vi "Lab Panel V5.11.vi"() -> ()   [LabVIEW 2013] (continued)
                            n2200 = Bundle(cluster=w3959, "amps"=w3963, "volts"=w3962, "pf"=w3961) -> (w3960:cluster{"amps":dbl, "volts":dbl, "pf":dbl})
                            n2201 = local write "ON L01-2"(w3960) -> ()
                          }
                        }
                      }
                      frame #1 {
                        n2202 = Unbundle(w3968) -> ("amps"=w3967:dbl, "volts"=w3966:dbl, "pf"=w3965:dbl)
                        n2203 = case shown="True" w3969 {
                          tunnel: w3976 -> [_ w4008]
                          tunnel: w3975 -> [_ w4015]
                          tunnel: w3974 -> [_ _]
                          tunnel: w3973 -> [_ _]
                          tunnel: w3972 -> [_ w4014]
                          tunnel: w3971 -> [_ w4013]
                          tunnel: w3970 -> [_ w3978]
                          tunnel: w3967 -> [_ w4010]
                          tunnel: w3966 -> [_ w4009]
                          tunnel: w3965 -> [_ w4007]
                          tunnel: w3964 -> [_ w3999]
                          frame False {
                          }
                          frame True {
                            n2204 = local read "TDMS LAB01-2"() -> (w4012:refnum<k34>)
                            n2205 = Build Array(w4009) -> (w4004:dbl[])
                            n2206 = Build Array(w4007) -> (w4003:dbl[])
                            n2207 = Build Array(w4014) -> (w4002:dbl[])
                            n2208 = Build Array(w4015) -> (w4001:dbl[])
                            n2209 = Build Array(w4010) -> (w4006:dbl[])
                            n2210 = Build Array(w4008) -> (w4005:dbl[])
                            n2211 = Build Array(w4013) -> (w4000:dbl[])
                            n2212 = Build Array("AMPS ON", "AMPS OFF", "VOLTS", "PF", "TEMP Live", "TEMP Neut", "CYCLE") -> (w3983:string[])
                            n2213 = Bundle By Name("Y"=w4006, "t0"=w3999) -> (w3998:waveform(dbl))  [unwired: 1 in]
                            n2214 = Bundle By Name("Y"=w4005, "t0"=w3999) -> (w3997:waveform(dbl))  [unwired: 1 in]
                            n2215 = Bundle By Name("Y"=w4004, "t0"=w3999) -> (w3996:waveform(dbl))  [unwired: 1 in]
                            n2216 = Bundle By Name("Y"=w4003, "t0"=w3999) -> (w3995:waveform(dbl))  [unwired: 1 in]
                            n2217 = Bundle By Name("Y"=w4002, "t0"=w3999) -> (w3994:waveform(dbl))  [unwired: 1 in]
                            n2218 = Bundle By Name("Y"=w4001, "t0"=w3999) -> (w3993:waveform(dbl))  [unwired: 1 in]
                            n2219 = Bundle By Name("Y"=w4000, "t0"=w3999) -> (w3992:waveform(dbl))  [unwired: 1 in]
                            n2220 = Build Array(w3998, w3997, w3996, w3995, w3994, w3993, w3992) -> (w3991:waveform(dbl)[])
                            n2221 = TDMS Write(0:w4012, 5:"TEST VALUES", 7:w3983, 9:w3991) -> (4:w3982:refnum<k34>, 6:w3981:string, 15:w3980:errorcluster)  [unwired: 2 in, 1 out]
                            n2222 = TDMS Write(0:w3982, 5:w3981, 7:"TIME", 9:w3978, 11:w3980) -> (15:w3977:errorcluster)  [unwired: 1 in, 3 out]
                            n2223 = local write "data file error"(w3977) -> ()
                          }
                        }
                      }
                    }
                  }
                }
              }
              frame #2 {
                n2224 = case shown="True" w4016 {
                  tunnel: w4020 -> [_ w4025]
                  tunnel: w4019 -> [_ w4024]
                  tunnel: w4018 -> [_ w4022]
                  tunnel: w4017 -> [_ w4021]
                  frame False {
                  }
                  frame True {
                    n2225 = local read "DISP LAB02-1"() -> (w4026:T4)
                    n2226 = local read "SIG LAB02-1"() -> (w4027:T2)
                    n2227 = local read "ON L02-1"() -> (w4023:cluster{"amps":dbl, "volts":dbl, "pf":dbl})
                    n2228 = Unbundle(w4027) -> ("AMPS"=w4033:dbl, "VOLTS"=w4031:dbl, "PF"=w4030:dbl, "Tmp Live"=w4029:dbl, "Tmp Neut"=w4032:dbl)
                    n2229 = Unbundle(w4026) -> ("CYCLE"=w4028:dbl)  [unwired: 2 out]
                    n2230 = stacked-sequence {
                      tunnel: w4033 -> [w4037 w4056]
                      tunnel: w4032 -> [_ w4055]
                      tunnel: w4031 -> [w4036 w4054]
                      tunnel: w4030 -> [w4035 w4053]
                      tunnel: w4029 -> [_ w4052]
                      tunnel: w4028 -> [_ w4051]
                      tunnel: w4025 -> [_ w4050]
                      tunnel: w4024 -> [w4038 _]
                      tunnel: w4023 -> [w4034 w4048]
                      tunnel: w4022 -> [_ w4049]
                      tunnel: w4021 -> [_ w4044]
                      frame #0 {
                        n2231 = case shown="True" w4038 {
                          tunnel: w4037 -> [_ w4043]
                          tunnel: w4036 -> [_ w4042]
                          tunnel: w4035 -> [_ w4041]
                          tunnel: w4034 -> [_ w4039]
                          frame False {
                          }
                          frame True {
                            n2232 = Bundle(cluster=w4039, "amps"=w4043, "volts"=w4042, "pf"=w4041) -> (w4040:cluster{"amps":dbl, "volts":dbl, "pf":dbl})
                            n2233 = local write "ON L02-1"(w4040) -> ()
                          }
                        }
                      }
                      frame #1 {
                        n2234 = Unbundle(w4048) -> ("amps"=w4047:dbl, "volts"=w4046:dbl, "pf"=w4045:dbl)
                        n2235 = case shown="True" w4049 {
                          tunnel: w4056 -> [_ w4088]
                          tunnel: w4055 -> [_ w4095]
                          tunnel: w4054 -> [_ _]
                          tunnel: w4053 -> [_ _]
                          tunnel: w4052 -> [_ w4094]
                          tunnel: w4051 -> [_ w4093]
                          tunnel: w4050 -> [_ w4058]
                          tunnel: w4047 -> [_ w4090]
                          tunnel: w4046 -> [_ w4089]
                          tunnel: w4045 -> [_ w4087]
                          tunnel: w4044 -> [_ w4079]
                          frame False {
                          }
                          frame True {
                            n2236 = local read "TDMS LAB02-1"() -> (w4092:refnum<k34>)
                            n2237 = Build Array(w4089) -> (w4084:dbl[])
                            n2238 = Build Array(w4087) -> (w4083:dbl[])
                            n2239 = Build Array(w4094) -> (w4082:dbl[])
                            n2240 = Build Array(w4095) -> (w4081:dbl[])
                            n2241 = Build Array(w4090) -> (w4086:dbl[])
                            n2242 = Build Array(w4088) -> (w4085:dbl[])
                            n2243 = Build Array(w4093) -> (w4080:dbl[])
                            n2244 = Build Array("AMPS ON", "AMPS OFF", "VOLTS", "PF", "TEMP Live", "TEMP Neut", "CYCLE") -> (w4063:string[])
                            n2245 = Bundle By Name("Y"=w4086, "t0"=w4079) -> (w4078:waveform(dbl))  [unwired: 1 in]
                            n2246 = Bundle By Name("Y"=w4085, "t0"=w4079) -> (w4077:waveform(dbl))  [unwired: 1 in]
                            n2247 = Bundle By Name("Y"=w4084, "t0"=w4079) -> (w4076:waveform(dbl))  [unwired: 1 in]
                            n2248 = Bundle By Name("Y"=w4083, "t0"=w4079) -> (w4075:waveform(dbl))  [unwired: 1 in]
                            n2249 = Bundle By Name("Y"=w4082, "t0"=w4079) -> (w4074:waveform(dbl))  [unwired: 1 in]
                            n2250 = Bundle By Name("Y"=w4081, "t0"=w4079) -> (w4073:waveform(dbl))  [unwired: 1 in]
                            n2251 = Bundle By Name("Y"=w4080, "t0"=w4079) -> (w4072:waveform(dbl))  [unwired: 1 in]
                            n2252 = Build Array(w4078, w4077, w4076, w4075, w4074, w4073, w4072) -> (w4071:waveform(dbl)[])
                            n2253 = TDMS Write(0:w4092, 5:"TEST VALUES", 7:w4063, 9:w4071) -> (4:w4062:refnum<k34>, 6:w4061:string, 15:w4060:errorcluster)  [unwired: 2 in, 1 out]
                            n2254 = TDMS Write(0:w4062, 5:w4061, 7:"TIME", 9:w4058, 11:w4060) -> (15:w4057:errorcluster)  [unwired: 1 in, 3 out]
                            n2255 = local write "data file error"(w4057) -> ()
                          }
                        }
                      }
                    }
                  }
                }
              }
              frame #3 {
                n2256 = case shown="True" w4096 {
                  tunnel: w4100 -> [_ w4105]
                  tunnel: w4099 -> [_ w4104]
                  tunnel: w4098 -> [_ w4102]
                  tunnel: w4097 -> [_ w4101]
                  frame False {
                  }
                  frame True {
                    n2257 = local read "DISP LAB02-2"() -> (w4106:T4)
                    n2258 = local read "SIG LAB02-2"() -> (w4107:T2)
                    n2259 = local read "ON L02-2"() -> (w4103:cluster{"amps":dbl, "volts":dbl, "pf":dbl})
                    n2260 = Unbundle(w4107) -> ("AMPS"=w4113:dbl, "VOLTS"=w4111:dbl, "PF"=w4110:dbl, "Tmp Live"=w4109:dbl, "Tmp Neut"=w4112:dbl)
                    n2261 = Unbundle(w4106) -> ("CYCLE"=w4108:dbl)  [unwired: 2 out]
                    n2262 = stacked-sequence {
                      tunnel: w4113 -> [w4117 w4136]
                      tunnel: w4112 -> [_ w4135]
                      tunnel: w4111 -> [w4116 w4134]
                      tunnel: w4110 -> [w4115 w4133]
                      tunnel: w4109 -> [_ w4132]
                      tunnel: w4108 -> [_ w4131]
                      tunnel: w4105 -> [_ w4130]
                      tunnel: w4104 -> [w4118 _]
                      tunnel: w4103 -> [w4114 w4128]
                      tunnel: w4102 -> [_ w4129]
                      tunnel: w4101 -> [_ w4124]
                      frame #0 {
                        n2263 = case shown="True" w4118 {
                          tunnel: w4117 -> [_ w4123]
                          tunnel: w4116 -> [_ w4122]
                          tunnel: w4115 -> [_ w4121]
                          tunnel: w4114 -> [_ w4119]
                          frame False {
                          }
                          frame True {
                            n2264 = Bundle(cluster=w4119, "amps"=w4123, "volts"=w4122, "pf"=w4121) -> (w4120:cluster{"amps":dbl, "volts":dbl, "pf":dbl})
                            n2265 = local write "ON L02-2"(w4120) -> ()
                          }
                        }
                      }
                      frame #1 {
                        n2266 = Unbundle(w4128) -> ("amps"=w4127:dbl, "volts"=w4126:dbl, "pf"=w4125:dbl)
                        n2267 = case shown="True" w4129 {
                          tunnel: w4136 -> [_ w4168]
                          tunnel: w4135 -> [_ w4175]
                          tunnel: w4134 -> [_ _]
                          tunnel: w4133 -> [_ _]
                          tunnel: w4132 -> [_ w4174]
                          tunnel: w4131 -> [_ w4173]
                          tunnel: w4130 -> [_ w4138]
                          tunnel: w4127 -> [_ w4170]
                          tunnel: w4126 -> [_ w4169]
                          tunnel: w4125 -> [_ w4167]
                          tunnel: w4124 -> [_ w4159]
                          frame False {
                          }
                          frame True {
                            n2268 = local read "TDMS LAB02-2"() -> (w4172:refnum<k34>)
                            n2269 = Build Array(w4169) -> (w4164:dbl[])
                            n2270 = Build Array(w4167) -> (w4163:dbl[])
                            n2271 = Build Array(w4174) -> (w4162:dbl[])
                            n2272 = Build Array(w4175) -> (w4161:dbl[])
                            n2273 = Build Array(w4170) -> (w4166:dbl[])
                            n2274 = Build Array(w4168) -> (w4165:dbl[])
                            n2275 = Build Array(w4173) -> (w4160:dbl[])
                            n2276 = Build Array("AMPS ON", "AMPS OFF", "VOLTS", "PF", "TEMP Live", "TEMP Neut", "CYCLE") -> (w4143:string[])
                            n2277 = Bundle By Name("Y"=w4166, "t0"=w4159) -> (w4158:waveform(dbl))  [unwired: 1 in]
                            n2278 = Bundle By Name("Y"=w4165, "t0"=w4159) -> (w4157:waveform(dbl))  [unwired: 1 in]
                            n2279 = Bundle By Name("Y"=w4164, "t0"=w4159) -> (w4156:waveform(dbl))  [unwired: 1 in]
                            n2280 = Bundle By Name("Y"=w4163, "t0"=w4159) -> (w4155:waveform(dbl))  [unwired: 1 in]
                            n2281 = Bundle By Name("Y"=w4162, "t0"=w4159) -> (w4154:waveform(dbl))  [unwired: 1 in]
                            n2282 = Bundle By Name("Y"=w4161, "t0"=w4159) -> (w4153:waveform(dbl))  [unwired: 1 in]
                            n2283 = Bundle By Name("Y"=w4160, "t0"=w4159) -> (w4152:waveform(dbl))  [unwired: 1 in]
                            n2284 = Build Array(w4158, w4157, w4156, w4155, w4154, w4153, w4152) -> (w4151:waveform(dbl)[])
                            n2285 = TDMS Write(0:w4172, 5:"TEST VALUES", 7:w4143, 9:w4151) -> (4:w4142:refnum<k34>, 6:w4141:string, 15:w4140:errorcluster)  [unwired: 2 in, 1 out]
                            n2286 = TDMS Write(0:w4142, 5:w4141, 7:"TIME", 9:w4138, 11:w4140) -> (15:w4137:errorcluster)  [unwired: 1 in, 3 out]
                            n2287 = local write "data file error"(w4137) -> ()
                          }
                        }
                      }
                    }
                  }
                }
              }
              frame #4 {
                n2288 = case shown="True" w4176 {
                  tunnel: w4180 -> [_ w4185]
                  tunnel: w4179 -> [_ w4184]
                  tunnel: w4178 -> [_ w4182]
                  tunnel: w4177 -> [_ w4181]
                  frame False {
                  }
                  frame True {
                    n2289 = local read "DISP LAB03-1"() -> (w4186:T4)
                    n2290 = local read "SIG LAB03-1"() -> (w4187:T2)
                    n2291 = local read "ON L03-1"() -> (w4183:cluster{"amps":dbl, "volts":dbl, "pf":dbl})
                    n2292 = Unbundle(w4187) -> ("AMPS"=w4193:dbl, "VOLTS"=w4191:dbl, "PF"=w4190:dbl, "Tmp Live"=w4189:dbl, "Tmp Neut"=w4192:dbl)
                    n2293 = Unbundle(w4186) -> ("CYCLE"=w4188:dbl)  [unwired: 2 out]
                    n2294 = stacked-sequence {
                      tunnel: w4193 -> [w4197 w4216]
                      tunnel: w4192 -> [_ w4215]
                      tunnel: w4191 -> [w4196 w4214]
                      tunnel: w4190 -> [w4195 w4213]
                      tunnel: w4189 -> [_ w4212]
                      tunnel: w4188 -> [_ w4211]
                      tunnel: w4185 -> [_ w4210]
                      tunnel: w4184 -> [w4198 _]
                      tunnel: w4183 -> [w4194 w4208]
                      tunnel: w4182 -> [_ w4209]
                      tunnel: w4181 -> [_ w4204]
                      frame #0 {
                        n2295 = case shown="True" w4198 {
                          tunnel: w4197 -> [_ w4203]
                          tunnel: w4196 -> [_ w4202]
                          tunnel: w4195 -> [_ w4201]
                          tunnel: w4194 -> [_ w4199]
                          frame False {
                          }
                          frame True {
                            n2296 = Bundle(cluster=w4199, "amps"=w4203, "volts"=w4202, "pf"=w4201) -> (w4200:cluster{"amps":dbl, "volts":dbl, "pf":dbl})
                            n2297 = local write "ON L03-1"(w4200) -> ()
                          }
                        }
                      }
                      frame #1 {
                        n2298 = Unbundle(w4208) -> ("amps"=w4207:dbl, "volts"=w4206:dbl, "pf"=w4205:dbl)
                        n2299 = case shown="True" w4209 {
                          tunnel: w4216 -> [_ w4248]
                          tunnel: w4215 -> [_ w4255]
                          tunnel: w4214 -> [_ _]
                          tunnel: w4213 -> [_ _]
                          tunnel: w4212 -> [_ w4254]
                          tunnel: w4211 -> [_ w4253]
                          tunnel: w4210 -> [_ w4218]
                          tunnel: w4207 -> [_ w4250]
                          tunnel: w4206 -> [_ w4249]
                          tunnel: w4205 -> [_ w4247]
                          tunnel: w4204 -> [_ w4239]
                          frame False {
                          }
                          frame True {
                            n2300 = local read "TDMS LAB03-1"() -> (w4252:refnum<k34>)
                            n2301 = Build Array(w4249) -> (w4244:dbl[])
                            n2302 = Build Array(w4247) -> (w4243:dbl[])
                            n2303 = Build Array(w4254) -> (w4242:dbl[])
                            n2304 = Build Array(w4255) -> (w4241:dbl[])
                            n2305 = Build Array(w4250) -> (w4246:dbl[])
                            n2306 = Build Array(w4248) -> (w4245:dbl[])
                            n2307 = Build Array(w4253) -> (w4240:dbl[])
                            n2308 = Build Array("AMPS ON", "AMPS OFF", "VOLTS", "PF", "TEMP Live", "TEMP Neut", "CYCLE") -> (w4223:string[])
                            n2309 = Bundle By Name("Y"=w4246, "t0"=w4239) -> (w4238:waveform(dbl))  [unwired: 1 in]
                            n2310 = Bundle By Name("Y"=w4245, "t0"=w4239) -> (w4237:waveform(dbl))  [unwired: 1 in]
                            n2311 = Bundle By Name("Y"=w4244, "t0"=w4239) -> (w4236:waveform(dbl))  [unwired: 1 in]
                            n2312 = Bundle By Name("Y"=w4243, "t0"=w4239) -> (w4235:waveform(dbl))  [unwired: 1 in]
                            n2313 = Bundle By Name("Y"=w4242, "t0"=w4239) -> (w4234:waveform(dbl))  [unwired: 1 in]
                            n2314 = Bundle By Name("Y"=w4241, "t0"=w4239) -> (w4233:waveform(dbl))  [unwired: 1 in]
                            n2315 = Bundle By Name("Y"=w4240, "t0"=w4239) -> (w4232:waveform(dbl))  [unwired: 1 in]
                            n2316 = Build Array(w4238, w4237, w4236, w4235, w4234, w4233, w4232) -> (w4231:waveform(dbl)[])
                            n2317 = TDMS Write(0:w4252, 5:"TEST VALUES", 7:w4223, 9:w4231) -> (4:w4222:refnum<k34>, 6:w4221:string, 15:w4220:errorcluster)  [unwired: 2 in, 1 out]
                            n2318 = TDMS Write(0:w4222, 5:w4221, 7:"TIME", 9:w4218, 11:w4220) -> (15:w4217:errorcluster)  [unwired: 1 in, 3 out]
                            n2319 = local write "data file error"(w4217) -> ()
                          }
                        }
                      }
                    }
                  }
                }
              }
              frame #5 {
                n2320 = case shown="True" w4256 {
                  tunnel: w4260 -> [_ w4265]
                  tunnel: w4259 -> [_ w4264]
                  tunnel: w4258 -> [_ w4262]
                  tunnel: w4257 -> [_ w4261]
                  frame False {
                  }
                  frame True {
                    n2321 = local read "DISP LAB03-2"() -> (w4266:T4)
                    n2322 = local read "SIG LAB03-2"() -> (w4267:T2)
                    n2323 = local read "ON L03-2"() -> (w4263:cluster{"amps":dbl, "volts":dbl, "pf":dbl})
                    n2324 = Unbundle(w4267) -> ("AMPS"=w4273:dbl, "VOLTS"=w4271:dbl, "PF"=w4270:dbl, "Tmp Live"=w4269:dbl, "Tmp Neut"=w4272:dbl)
                    n2325 = Unbundle(w4266) -> ("CYCLE"=w4268:dbl)  [unwired: 2 out]
                    n2326 = stacked-sequence {
                      tunnel: w4273 -> [w4277 w4296]
                      tunnel: w4272 -> [_ w4295]
                      tunnel: w4271 -> [w4276 w4294]
                      tunnel: w4270 -> [w4275 w4293]
                      tunnel: w4269 -> [_ w4292]
                      tunnel: w4268 -> [_ w4291]
                      tunnel: w4265 -> [_ w4290]
                      tunnel: w4264 -> [w4278 _]
                      tunnel: w4263 -> [w4274 w4288]
                      tunnel: w4262 -> [_ w4289]
                      tunnel: w4261 -> [_ w4284]
                      frame #0 {
                        n2327 = case shown="True" w4278 {
                          tunnel: w4277 -> [_ w4283]
                          tunnel: w4276 -> [_ w4282]
                          tunnel: w4275 -> [_ w4281]
                          tunnel: w4274 -> [_ w4279]
                          frame False {
                          }
                          frame True {
                            n2328 = Bundle(cluster=w4279, "amps"=w4283, "volts"=w4282, "pf"=w4281) -> (w4280:cluster{"amps":dbl, "volts":dbl, "pf":dbl})
                            n2329 = local write "ON L03-2"(w4280) -> ()
                          }
                        }
                      }
                      frame #1 {
                        n2330 = Unbundle(w4288) -> ("amps"=w4287:dbl, "volts"=w4286:dbl, "pf"=w4285:dbl)
                        n2331 = case shown="True" w4289 {
                          tunnel: w4296 -> [_ w4328]
                          tunnel: w4295 -> [_ w4335]
                          tunnel: w4294 -> [_ _]
                          tunnel: w4293 -> [_ _]
                          tunnel: w4292 -> [_ w4334]
                          tunnel: w4291 -> [_ w4333]
                          tunnel: w4290 -> [_ w4298]
                          tunnel: w4287 -> [_ w4330]
                          tunnel: w4286 -> [_ w4329]
                          tunnel: w4285 -> [_ w4327]
                          tunnel: w4284 -> [_ w4319]
                          frame False {
                          }
                          frame True {
                            n2332 = local read "TDMS LAB03-2"() -> (w4332:refnum<k34>)
                            n2333 = Build Array(w4329) -> (w4324:dbl[])
                            n2334 = Build Array(w4327) -> (w4323:dbl[])
                            n2335 = Build Array(w4334) -> (w4322:dbl[])
                            n2336 = Build Array(w4335) -> (w4321:dbl[])
                            n2337 = Build Array(w4330) -> (w4326:dbl[])
                            n2338 = Build Array(w4328) -> (w4325:dbl[])
                            n2339 = Build Array(w4333) -> (w4320:dbl[])
                            n2340 = Build Array("AMPS ON", "AMPS OFF", "VOLTS", "PF", "TEMP Live", "TEMP Neut", "CYCLE") -> (w4303:string[])
                            n2341 = Bundle By Name("Y"=w4326, "t0"=w4319) -> (w4318:waveform(dbl))  [unwired: 1 in]
                            n2342 = Bundle By Name("Y"=w4325, "t0"=w4319) -> (w4317:waveform(dbl))  [unwired: 1 in]
                            n2343 = Bundle By Name("Y"=w4324, "t0"=w4319) -> (w4316:waveform(dbl))  [unwired: 1 in]
                            n2344 = Bundle By Name("Y"=w4323, "t0"=w4319) -> (w4315:waveform(dbl))  [unwired: 1 in]
                            n2345 = Bundle By Name("Y"=w4322, "t0"=w4319) -> (w4314:waveform(dbl))  [unwired: 1 in]
                            n2346 = Bundle By Name("Y"=w4321, "t0"=w4319) -> (w4313:waveform(dbl))  [unwired: 1 in]
                            n2347 = Bundle By Name("Y"=w4320, "t0"=w4319) -> (w4312:waveform(dbl))  [unwired: 1 in]
                            n2348 = Build Array(w4318, w4317, w4316, w4315, w4314, w4313, w4312) -> (w4311:waveform(dbl)[])
                            n2349 = TDMS Write(0:w4332, 5:"TEST VALUES", 7:w4303, 9:w4311) -> (4:w4302:refnum<k34>, 6:w4301:string, 15:w4300:errorcluster)  [unwired: 2 in, 1 out]
                            n2350 = TDMS Write(0:w4302, 5:w4301, 7:"TIME", 9:w4298, 11:w4300) -> (15:w4297:errorcluster)  [unwired: 1 in, 3 out]
                            n2351 = local write "data file error"(w4297) -> ()
                          }
                        }
                      }
                    }
                  }
                }
              }
              frame #6 {
                n2352 = case shown="True" w4336 {
                  tunnel: w4340 -> [_ w4345]
                  tunnel: w4339 -> [_ w4344]
                  tunnel: w4338 -> [_ w4342]
                  tunnel: w4337 -> [_ w4341]
                  frame False {
                  }
                  frame True {
                    n2353 = local read "DISP LAB04-1"() -> (w4346:T4)
                    n2354 = local read "SIG LAB04-1"() -> (w4347:T2)
                    n2355 = local read "ON L04-1"() -> (w4343:cluster{"amps":dbl, "volts":dbl, "pf":dbl})
                    n2356 = Unbundle(w4347) -> ("AMPS"=w4353:dbl, "VOLTS"=w4351:dbl, "PF"=w4350:dbl, "Tmp Live"=w4349:dbl, "Tmp Neut"=w4352:dbl)
                    n2357 = Unbundle(w4346) -> ("CYCLE"=w4348:dbl)  [unwired: 2 out]
                    n2358 = stacked-sequence {
                      tunnel: w4353 -> [w4357 w4376]
                      tunnel: w4352 -> [_ w4375]
                      tunnel: w4351 -> [w4356 w4374]
                      tunnel: w4350 -> [w4355 w4373]
                      tunnel: w4349 -> [_ w4372]
                      tunnel: w4348 -> [_ w4371]
                      tunnel: w4345 -> [_ w4370]
                      tunnel: w4344 -> [w4358 _]
                      tunnel: w4343 -> [w4354 w4368]
                      tunnel: w4342 -> [_ w4369]
                      tunnel: w4341 -> [_ w4364]
                      frame #0 {
                        n2359 = case shown="True" w4358 {
                          tunnel: w4357 -> [_ w4363]
                          tunnel: w4356 -> [_ w4362]
                          tunnel: w4355 -> [_ w4361]
                          tunnel: w4354 -> [_ w4359]
                          frame False {
                          }
                          frame True {
                            n2360 = Bundle(cluster=w4359, "amps"=w4363, "volts"=w4362, "pf"=w4361) -> (w4360:cluster{"amps":dbl, "volts":dbl, "pf":dbl})
                            n2361 = local write "ON L04-1"(w4360) -> ()
                          }
                        }
                      }
                      frame #1 {
                        n2362 = Unbundle(w4368) -> ("amps"=w4367:dbl, "volts"=w4366:dbl, "pf"=w4365:dbl)
                        n2363 = case shown="True" w4369 {
                          tunnel: w4376 -> [_ w4408]
                          tunnel: w4375 -> [_ w4415]
                          tunnel: w4374 -> [_ _]
                          tunnel: w4373 -> [_ _]
                          tunnel: w4372 -> [_ w4414]
                          tunnel: w4371 -> [_ w4413]
                          tunnel: w4370 -> [_ w4378]
                          tunnel: w4367 -> [_ w4410]
                          tunnel: w4366 -> [_ w4409]
                          tunnel: w4365 -> [_ w4407]
                          tunnel: w4364 -> [_ w4399]
                          frame False {
                          }
                          frame True {
                            n2364 = local read "TDMS LAB04-1"() -> (w4412:refnum<k34>)
                            n2365 = Build Array(w4409) -> (w4404:dbl[])
                            n2366 = Build Array(w4407) -> (w4403:dbl[])
                            n2367 = Build Array(w4414) -> (w4402:dbl[])
                            n2368 = Build Array(w4415) -> (w4401:dbl[])
                            n2369 = Build Array(w4410) -> (w4406:dbl[])
                            n2370 = Build Array(w4408) -> (w4405:dbl[])
                            n2371 = Build Array(w4413) -> (w4400:dbl[])
                            n2372 = Build Array("AMPS ON", "AMPS OFF", "VOLTS", "PF", "TEMP Live", "TEMP Neut", "CYCLE") -> (w4383:string[])
                            n2373 = Bundle By Name("Y"=w4406, "t0"=w4399) -> (w4398:waveform(dbl))  [unwired: 1 in]
                            n2374 = Bundle By Name("Y"=w4405, "t0"=w4399) -> (w4397:waveform(dbl))  [unwired: 1 in]
                            n2375 = Bundle By Name("Y"=w4404, "t0"=w4399) -> (w4396:waveform(dbl))  [unwired: 1 in]
                            n2376 = Bundle By Name("Y"=w4403, "t0"=w4399) -> (w4395:waveform(dbl))  [unwired: 1 in]
                            n2377 = Bundle By Name("Y"=w4402, "t0"=w4399) -> (w4394:waveform(dbl))  [unwired: 1 in]
                            n2378 = Bundle By Name("Y"=w4401, "t0"=w4399) -> (w4393:waveform(dbl))  [unwired: 1 in]
                            n2379 = Bundle By Name("Y"=w4400, "t0"=w4399) -> (w4392:waveform(dbl))  [unwired: 1 in]
                            n2380 = Build Array(w4398, w4397, w4396, w4395, w4394, w4393, w4392) -> (w4391:waveform(dbl)[])
                            n2381 = TDMS Write(0:w4412, 5:"TEST VALUES", 7:w4383, 9:w4391) -> (4:w4382:refnum<k34>, 6:w4381:string, 15:w4380:errorcluster)  [unwired: 2 in, 1 out]
                            n2382 = TDMS Write(0:w4382, 5:w4381, 7:"TIME", 9:w4378, 11:w4380) -> (15:w4377:errorcluster)  [unwired: 1 in, 3 out]
                            n2383 = local write "data file error"(w4377) -> ()
                          }
                        }
                      }
                    }
                  }
                }
              }
              frame #7 {
                n2384 = case shown="True" w4416 {
                  tunnel: w4420 -> [_ w4425]
                  tunnel: w4419 -> [_ w4424]
                  tunnel: w4418 -> [_ w4422]
                  tunnel: w4417 -> [_ w4421]
                  frame False {
                  }
                  frame True {
                    n2385 = local read "DISP LAB04-2"() -> (w4426:T4)
                    n2386 = local read "SIG LAB04-2"() -> (w4427:T2)
                    n2387 = local read "ON L04-2"() -> (w4423:cluster{"amps":dbl, "volts":dbl, "pf":dbl})
                    n2388 = Unbundle(w4427) -> ("AMPS"=w4433:dbl, "VOLTS"=w4431:dbl, "PF"=w4430:dbl, "Tmp Live"=w4429:dbl, "Tmp Neut"=w4432:dbl)
                    n2389 = Unbundle(w4426) -> ("CYCLE"=w4428:dbl)  [unwired: 2 out]
                    n2390 = stacked-sequence {
                      tunnel: w4433 -> [w4437 w4456]
                      tunnel: w4432 -> [_ w4455]
                      tunnel: w4431 -> [w4436 w4454]
                      tunnel: w4430 -> [w4435 w4453]
                      tunnel: w4429 -> [_ w4452]
                      tunnel: w4428 -> [_ w4451]
                      tunnel: w4425 -> [_ w4450]
                      tunnel: w4424 -> [w4438 _]
                      tunnel: w4423 -> [w4434 w4448]
                      tunnel: w4422 -> [_ w4449]
                      tunnel: w4421 -> [_ w4444]
                      frame #0 {
                        n2391 = case shown="True" w4438 {
                          tunnel: w4437 -> [_ w4443]
                          tunnel: w4436 -> [_ w4442]
                          tunnel: w4435 -> [_ w4441]
                          tunnel: w4434 -> [_ w4439]
                          frame False {
                          }
                          frame True {
                            n2392 = Bundle(cluster=w4439, "amps"=w4443, "volts"=w4442, "pf"=w4441) -> (w4440:cluster{"amps":dbl, "volts":dbl, "pf":dbl})
                            n2393 = local write "ON L04-2"(w4440) -> ()
                          }
                        }
                      }
                      frame #1 {
                        n2394 = Unbundle(w4448) -> ("amps"=w4447:dbl, "volts"=w4446:dbl, "pf"=w4445:dbl)
                        n2395 = case shown="True" w4449 {
                          tunnel: w4456 -> [_ w4488]
                          tunnel: w4455 -> [_ w4495]
                          tunnel: w4454 -> [_ _]
                          tunnel: w4453 -> [_ _]
                          tunnel: w4452 -> [_ w4494]
                          tunnel: w4451 -> [_ w4493]
                          tunnel: w4450 -> [_ w4458]
                          tunnel: w4447 -> [_ w4490]
                          tunnel: w4446 -> [_ w4489]
                          tunnel: w4445 -> [_ w4487]
                          tunnel: w4444 -> [_ w4479]
                          frame False {
                          }
                          frame True {
                            n2396 = local read "TDMS LAB04-2"() -> (w4492:refnum<k34>)
                            n2397 = Build Array(w4489) -> (w4484:dbl[])
                            n2398 = Build Array(w4487) -> (w4483:dbl[])
                            n2399 = Build Array(w4494) -> (w4482:dbl[])
                            n2400 = Build Array(w4495) -> (w4481:dbl[])
                            n2401 = Build Array(w4490) -> (w4486:dbl[])
                            n2402 = Build Array(w4488) -> (w4485:dbl[])
                            n2403 = Build Array(w4493) -> (w4480:dbl[])
                            n2404 = Build Array("AMPS ON", "AMPS OFF", "VOLTS", "PF", "TEMP Live", "TEMP Neut", "CYCLE") -> (w4463:string[])
                            n2405 = Bundle By Name("Y"=w4486, "t0"=w4479) -> (w4478:waveform(dbl))  [unwired: 1 in]
                            n2406 = Bundle By Name("Y"=w4485, "t0"=w4479) -> (w4477:waveform(dbl))  [unwired: 1 in]
                            n2407 = Bundle By Name("Y"=w4484, "t0"=w4479) -> (w4476:waveform(dbl))  [unwired: 1 in]
                            n2408 = Bundle By Name("Y"=w4483, "t0"=w4479) -> (w4475:waveform(dbl))  [unwired: 1 in]
                            n2409 = Bundle By Name("Y"=w4482, "t0"=w4479) -> (w4474:waveform(dbl))  [unwired: 1 in]
                            n2410 = Bundle By Name("Y"=w4481, "t0"=w4479) -> (w4473:waveform(dbl))  [unwired: 1 in]
                            n2411 = Bundle By Name("Y"=w4480, "t0"=w4479) -> (w4472:waveform(dbl))  [unwired: 1 in]
                            n2412 = Build Array(w4478, w4477, w4476, w4475, w4474, w4473, w4472) -> (w4471:waveform(dbl)[])
                            n2413 = TDMS Write(0:w4492, 5:"TEST VALUES", 7:w4463, 9:w4471) -> (4:w4462:refnum<k34>, 6:w4461:string, 15:w4460:errorcluster)  [unwired: 2 in, 1 out]
                            n2414 = TDMS Write(0:w4462, 5:w4461, 7:"TIME", 9:w4458, 11:w4460) -> (15:w4457:errorcluster)  [unwired: 1 in, 3 out]
                            n2415 = local write "data file error"(w4457) -> ()
                          }
                        }
                      }
                    }
                  }
                }
              }
              frame #8 {
                n2416 = case shown="True" w4496 {
                  tunnel: w4500 -> [_ w4505]
                  tunnel: w4499 -> [_ w4504]
                  tunnel: w4498 -> [_ w4502]
                  tunnel: w4497 -> [_ w4501]
                  frame False {
                  }
                  frame True {
                    n2417 = local read "DISP LAB05-1"() -> (w4506:T4)
                    n2418 = local read "SIG LAB05-1"() -> (w4507:T2)
                    n2419 = local read "ON L05-1"() -> (w4503:cluster{"amps":dbl, "volts":dbl, "pf":dbl})
                    n2420 = Unbundle(w4507) -> ("AMPS"=w4513:dbl, "VOLTS"=w4511:dbl, "PF"=w4510:dbl, "Tmp Live"=w4509:dbl, "Tmp Neut"=w4512:dbl)
                    n2421 = Unbundle(w4506) -> ("CYCLE"=w4508:dbl)  [unwired: 2 out]
                    n2422 = stacked-sequence {
                      tunnel: w4513 -> [w4517 w4536]
                      tunnel: w4512 -> [_ w4535]
                      tunnel: w4511 -> [w4516 w4534]
                      tunnel: w4510 -> [w4515 w4533]
                      tunnel: w4509 -> [_ w4532]
                      tunnel: w4508 -> [_ w4531]
                      tunnel: w4505 -> [_ w4530]
                      tunnel: w4504 -> [w4518 _]
                      tunnel: w4503 -> [w4514 w4528]
                      tunnel: w4502 -> [_ w4529]
                      tunnel: w4501 -> [_ w4524]
                      frame #0 {
                        n2423 = case shown="True" w4518 {
                          tunnel: w4517 -> [_ w4523]
                          tunnel: w4516 -> [_ w4522]
                          tunnel: w4515 -> [_ w4521]
                          tunnel: w4514 -> [_ w4519]
                          frame False {
                          }
                          frame True {
                            n2424 = Bundle(cluster=w4519, "amps"=w4523, "volts"=w4522, "pf"=w4521) -> (w4520:cluster{"amps":dbl, "volts":dbl, "pf":dbl})
                            n2425 = local write "ON L05-1"(w4520) -> ()
                          }
                        }
                      }
                      frame #1 {
                        n2426 = Unbundle(w4528) -> ("amps"=w4527:dbl, "volts"=w4526:dbl, "pf"=w4525:dbl)
                        n2427 = case shown="True" w4529 {
                          tunnel: w4536 -> [_ w4568]
                          tunnel: w4535 -> [_ w4575]
                          tunnel: w4534 -> [_ _]
                          tunnel: w4533 -> [_ _]
                          tunnel: w4532 -> [_ w4574]
                          tunnel: w4531 -> [_ w4573]
                          tunnel: w4530 -> [_ w4538]
                          tunnel: w4527 -> [_ w4570]
                          tunnel: w4526 -> [_ w4569]
                          tunnel: w4525 -> [_ w4567]
                          tunnel: w4524 -> [_ w4559]
                          frame False {
                          }
                          frame True {
                            n2428 = local read "TDMS LAB05-1"() -> (w4572:refnum<k34>)
                            n2429 = Build Array(w4569) -> (w4564:dbl[])
                            n2430 = Build Array(w4567) -> (w4563:dbl[])
                            n2431 = Build Array(w4574) -> (w4562:dbl[])
                            n2432 = Build Array(w4575) -> (w4561:dbl[])
                            n2433 = Build Array(w4570) -> (w4566:dbl[])
                            n2434 = Build Array(w4568) -> (w4565:dbl[])
                            n2435 = Build Array(w4573) -> (w4560:dbl[])
                            n2436 = Build Array("AMPS ON", "AMPS OFF", "VOLTS", "PF", "TEMP Live", "TEMP Neut", "CYCLE") -> (w4543:string[])
                            n2437 = Bundle By Name("Y"=w4566, "t0"=w4559) -> (w4558:waveform(dbl))  [unwired: 1 in]
                            n2438 = Bundle By Name("Y"=w4565, "t0"=w4559) -> (w4557:waveform(dbl))  [unwired: 1 in]
                            n2439 = Bundle By Name("Y"=w4564, "t0"=w4559) -> (w4556:waveform(dbl))  [unwired: 1 in]
                            n2440 = Bundle By Name("Y"=w4563, "t0"=w4559) -> (w4555:waveform(dbl))  [unwired: 1 in]
                            n2441 = Bundle By Name("Y"=w4562, "t0"=w4559) -> (w4554:waveform(dbl))  [unwired: 1 in]
                            n2442 = Bundle By Name("Y"=w4561, "t0"=w4559) -> (w4553:waveform(dbl))  [unwired: 1 in]
                            n2443 = Bundle By Name("Y"=w4560, "t0"=w4559) -> (w4552:waveform(dbl))  [unwired: 1 in]
                            n2444 = Build Array(w4558, w4557, w4556, w4555, w4554, w4553, w4552) -> (w4551:waveform(dbl)[])
                            n2445 = TDMS Write(0:w4572, 5:"TEST VALUES", 7:w4543, 9:w4551) -> (4:w4542:refnum<k34>, 6:w4541:string, 15:w4540:errorcluster)  [unwired: 2 in, 1 out]
                            n2446 = TDMS Write(0:w4542, 5:w4541, 7:"TIME", 9:w4538, 11:w4540) -> (15:w4537:errorcluster)  [unwired: 1 in, 3 out]
                            n2447 = local write "data file error"(w4537) -> ()
                          }
                        }
                      }
                    }
                  }
                }
              }
              frame #9 {
                n2448 = case shown="True" w4576 {
                  tunnel: w4580 -> [_ w4585]
                  tunnel: w4579 -> [_ w4584]
                  tunnel: w4578 -> [_ w4582]
                  tunnel: w4577 -> [_ w4581]
                  frame False {
                  }
                  frame True {
                    n2449 = local read "DISP LAB05-2"() -> (w4586:T4)
                    n2450 = local read "SIG LAB05-2"() -> (w4587:T2)
                    n2451 = local read "ON L05-2"() -> (w4583:cluster{"amps":dbl, "volts":dbl, "pf":dbl})
                    n2452 = Unbundle(w4587) -> ("AMPS"=w4593:dbl, "VOLTS"=w4591:dbl, "PF"=w4590:dbl, "Tmp Live"=w4589:dbl, "Tmp Neut"=w4592:dbl)
                    n2453 = Unbundle(w4586) -> ("CYCLE"=w4588:dbl)  [unwired: 2 out]
                    n2454 = stacked-sequence {
                      tunnel: w4593 -> [w4597 w4616]
                      tunnel: w4592 -> [_ w4615]
                      tunnel: w4591 -> [w4596 w4614]
                      tunnel: w4590 -> [w4595 w4613]
                      tunnel: w4589 -> [_ w4612]
                      tunnel: w4588 -> [_ w4611]
                      tunnel: w4585 -> [_ w4610]
                      tunnel: w4584 -> [w4598 _]
                      tunnel: w4583 -> [w4594 w4608]
                      tunnel: w4582 -> [_ w4609]
                      tunnel: w4581 -> [_ w4604]
                      frame #0 {
                        n2455 = case shown="True" w4598 {
                          tunnel: w4597 -> [_ w4603]
                          tunnel: w4596 -> [_ w4602]
                          tunnel: w4595 -> [_ w4601]
                          tunnel: w4594 -> [_ w4599]
                          frame False {
                          }
                          frame True {
                            n2456 = Bundle(cluster=w4599, "amps"=w4603, "volts"=w4602, "pf"=w4601) -> (w4600:cluster{"amps":dbl, "volts":dbl, "pf":dbl})
                            n2457 = local write "ON L05-2"(w4600) -> ()
                          }
                        }
                      }
                      frame #1 {
                        n2458 = Unbundle(w4608) -> ("amps"=w4607:dbl, "volts"=w4606:dbl, "pf"=w4605:dbl)
                        n2459 = case shown="True" w4609 {
                          tunnel: w4616 -> [_ w4648]
                          tunnel: w4615 -> [_ w4655]
                          tunnel: w4614 -> [_ _]
                          tunnel: w4613 -> [_ _]
                          tunnel: w4612 -> [_ w4654]
                          tunnel: w4611 -> [_ w4653]
                          tunnel: w4610 -> [_ w4618]
                          tunnel: w4607 -> [_ w4650]
                          tunnel: w4606 -> [_ w4649]
                          tunnel: w4605 -> [_ w4647]
                          tunnel: w4604 -> [_ w4639]
                          frame False {
                          }
                          frame True {
                            n2460 = local read "TDMS LAB05-2"() -> (w4652:refnum<k34>)
                            n2461 = Build Array(w4649) -> (w4644:dbl[])
                            n2462 = Build Array(w4647) -> (w4643:dbl[])
                            n2463 = Build Array(w4654) -> (w4642:dbl[])
                            n2464 = Build Array(w4655) -> (w4641:dbl[])
                            n2465 = Build Array(w4650) -> (w4646:dbl[])
                            n2466 = Build Array(w4648) -> (w4645:dbl[])
                            n2467 = Build Array(w4653) -> (w4640:dbl[])
                            n2468 = Build Array("AMPS ON", "AMPS OFF", "VOLTS", "PF", "TEMP Live", "TEMP Neut", "CYCLE") -> (w4623:string[])
                            n2469 = Bundle By Name("Y"=w4646, "t0"=w4639) -> (w4638:waveform(dbl))  [unwired: 1 in]
                            n2470 = Bundle By Name("Y"=w4645, "t0"=w4639) -> (w4637:waveform(dbl))  [unwired: 1 in]
                            n2471 = Bundle By Name("Y"=w4644, "t0"=w4639) -> (w4636:waveform(dbl))  [unwired: 1 in]
                            n2472 = Bundle By Name("Y"=w4643, "t0"=w4639) -> (w4635:waveform(dbl))  [unwired: 1 in]
                            n2473 = Bundle By Name("Y"=w4642, "t0"=w4639) -> (w4634:waveform(dbl))  [unwired: 1 in]
                            n2474 = Bundle By Name("Y"=w4641, "t0"=w4639) -> (w4633:waveform(dbl))  [unwired: 1 in]
                            n2475 = Bundle By Name("Y"=w4640, "t0"=w4639) -> (w4632:waveform(dbl))  [unwired: 1 in]
                            n2476 = Build Array(w4638, w4637, w4636, w4635, w4634, w4633, w4632) -> (w4631:waveform(dbl)[])
                            n2477 = TDMS Write(0:w4652, 5:"TEST VALUES", 7:w4623, 9:w4631) -> (4:w4622:refnum<k34>, 6:w4621:string, 15:w4620:errorcluster)  [unwired: 2 in, 1 out]
                            n2478 = TDMS Write(0:w4622, 5:w4621, 7:"TIME", 9:w4618, 11:w4620) -> (15:w4617:errorcluster)  [unwired: 1 in, 3 out]
                            n2479 = local write "data file error"(w4617) -> ()
                          }
                        }
                      }
                    }
                  }
                }
              }
            }
          }
          frame #13 {
            # "display test values on chart"
            n2480 = local read "jig cycle"() -> (w4660:dbl)
            n2481 = local read "on loops"() -> (w4662:dbl)
            n2482 = Add(x=w4662, y=2) -> (x+y=w4659:dbl)
            n2483 = Equal?(x=w4660, y=1) -> (x = y?=w4658:bool)
            n2484 = Equal?(x=w4660, y=w4659) -> (x = y?=w4657:bool)
            n2485 = Or(x=w4658, y=w4657) -> (x .or. y?=w4656:bool)
            "graph flag" <- w4656
            n2486 = global write "Global display 3.vi" "graph flag"(w4656) -> ()
            n2487 = case shown="True" w4656 {
              frame False {
              }
              frame True {
                n2488 = local read "SIG LAB05-1"() -> (w4705:T2)
                n2489 = local read "SIG LAB04-2"() -> (w4706:T2)
                n2490 = local read "SIG LAB05-2"() -> (w4704:T2)
                n2491 = local read "SIG LAB04-1"() -> (w4707:T2)
                n2492 = local read "SIG LAB03-1"() -> (w4709:T2)
                n2493 = local read "SIG LAB03-2"() -> (w4708:T2)
                n2494 = local read "SIG LAB01-1"() -> (w4713:T2)
                n2495 = local read "SIG LAB02-2"() -> (w4710:T2)
                n2496 = local read "SIG LAB02-1"() -> (w4711:T2)
                n2497 = local read "SIG LAB01-2"() -> (w4712:T2)
                n2498 = Unbundle(w4706) -> ("AMPS"=w4696:dbl, "VOLTS"=w4686:dbl, "Tmp Live"=w4676:dbl, "Tmp Neut"=w4666:dbl)  [unwired: 1 out]
                n2499 = Unbundle(w4705) -> ("AMPS"=w4695:dbl, "VOLTS"=w4685:dbl, "Tmp Live"=w4675:dbl, "Tmp Neut"=w4665:dbl)  [unwired: 1 out]
                n2500 = Unbundle(w4704) -> ("AMPS"=w4694:dbl, "VOLTS"=w4684:dbl, "Tmp Live"=w4674:dbl, "Tmp Neut"=w4664:dbl)  [unwired: 1 out]
                n2501 = Unbundle(w4707) -> ("AMPS"=w4697:dbl, "VOLTS"=w4687:dbl, "Tmp Live"=w4677:dbl, "Tmp Neut"=w4667:dbl)  [unwired: 1 out]
                n2502 = Unbundle(w4708) -> ("AMPS"=w4698:dbl, "VOLTS"=w4688:dbl, "Tmp Live"=w4678:dbl, "Tmp Neut"=w4668:dbl)  [unwired: 1 out]
                n2503 = Unbundle(w4709) -> ("AMPS"=w4699:dbl, "VOLTS"=w4689:dbl, "Tmp Live"=w4679:dbl, "Tmp Neut"=w4669:dbl)  [unwired: 1 out]
                n2504 = Unbundle(w4710) -> ("AMPS"=w4700:dbl, "VOLTS"=w4690:dbl, "Tmp Live"=w4680:dbl, "Tmp Neut"=w4670:dbl)  [unwired: 1 out]
                n2505 = Unbundle(w4711) -> ("AMPS"=w4701:dbl, "VOLTS"=w4691:dbl, "Tmp Live"=w4681:dbl, "Tmp Neut"=w4671:dbl)  [unwired: 1 out]
                n2506 = Unbundle(w4713) -> ("AMPS"=w4703:dbl, "VOLTS"=w4693:dbl, "Tmp Live"=w4683:dbl, "Tmp Neut"=w4673:dbl)  [unwired: 1 out]
                n2507 = Unbundle(w4712) -> ("AMPS"=w4702:dbl, "VOLTS"=w4692:dbl, "Tmp Live"=w4682:dbl, "Tmp Neut"=w4672:dbl)  [unwired: 1 out]
                n2508 = stacked-sequence {
                  tunnel: w4703 -> [w4745 _ _]
                  tunnel: w4702 -> [w4744 _ _]
                  tunnel: w4701 -> [w4735 _ _]
                  tunnel: w4700 -> [w4734 _ _]
                  tunnel: w4699 -> [w4724 _ _]
                  tunnel: w4698 -> [w4723 _ _]
                  tunnel: w4697 -> [_ w4768 _]
                  tunnel: w4696 -> [_ w4767 _]
                  tunnel: w4695 -> [_ w4757 _]
                  tunnel: w4694 -> [_ w4756 _]
                  tunnel: w4693 -> [w4742 _ _]
                  tunnel: w4692 -> [w4741 _ _]
                  tunnel: w4691 -> [w4732 _ _]
                  tunnel: w4690 -> [w4731 _ _]
                  tunnel: w4689 -> [w4722 _ _]
                  tunnel: w4688 -> [w4721 _ _]
                  tunnel: w4687 -> [_ w4766 _]
                  tunnel: w4686 -> [_ w4765 _]
                  tunnel: w4685 -> [_ w4755 _]
                  tunnel: w4684 -> [_ w4754 _]
                  tunnel: w4683 -> [w4739 _ _]
                  tunnel: w4682 -> [w4737 _ _]
                  tunnel: w4681 -> [w4728 _ _]
                  tunnel: w4680 -> [w4726 _ _]
                  tunnel: w4679 -> [w4720 _ _]
                  tunnel: w4678 -> [w4718 _ _]
                  tunnel: w4677 -> [_ w4764 _]
                  tunnel: w4676 -> [_ w4762 _]
                  tunnel: w4675 -> [_ w4753 _]
                  tunnel: w4674 -> [_ w4751 _]
                  tunnel: w4673 -> [w4738 _ _]
                  tunnel: w4672 -> [w4736 _ _]
                  tunnel: w4671 -> [w4727 _ _]
                  tunnel: w4670 -> [w4725 _ _]
                  tunnel: w4669 -> [w4719 _ _]
                  tunnel: w4668 -> [w4717 _ _]
                  tunnel: w4667 -> [_ w4763 _]
                  tunnel: w4666 -> [_ w4761 _]
                  tunnel: w4665 -> [_ w4752 _]
                  tunnel: w4664 -> [_ w4750 _]
